vi "SetMeasurement.vi"(1 "int32DeviceNumber":i32, 2 "MeassurementSettings":T3, 3 "FilterSettings":T2, 4 "TriggerSettings":T1) -> (0 "success":i32)   [LabVIEW 2009]
panel:
  in  "measurementFlag":u32
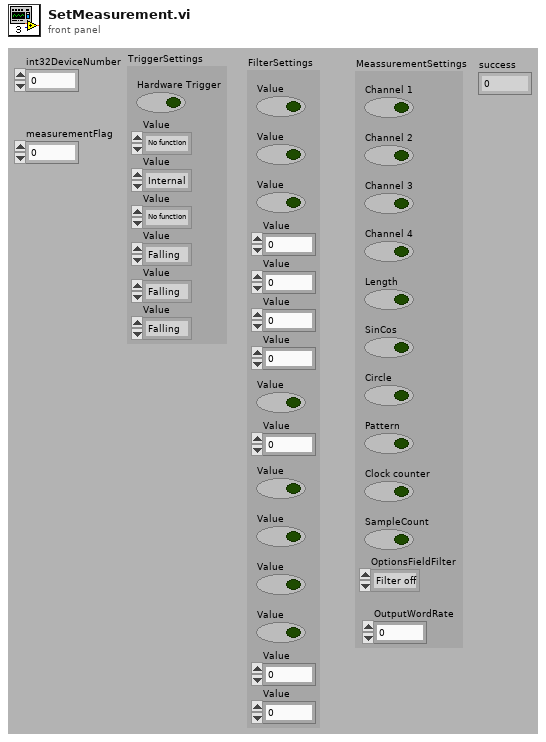
[diagram p1: front panel]
types:
  T1 = cluster{"Hardware Trigger":bool, "Value":enum32{"No function", "Start trigger", "Start/Stop trigger", "Start/Stop processed"}, "Value":enum32{"Internal", "External"}, "Value":enum32{"No function", "Single value"}, "Value":enum32{"Falling", "Rising"}, "Value":enum32{"Falling", "Rising"}, "Value":enum32{"Falling", "Rising"}}
  T2 = cluster{"Value":bool, "Value":bool, "Value":bool, "Value":dbl, "Value":dbl, "Value":dbl, "Value":dbl, "Value":bool, "Value":dbl, "Value":bool, "Value":bool, "Value":bool, "Value":bool, "Value":u8, "Value":u8}
  T3 = cluster{"Channel 1":bool, "Channel 2":bool, "Channel 3":bool, "Channel 4":bool, "Length":bool, "SinCos":bool, "Circle":bool, "Pattern":bool, "Clock counter":bool, "SampleCount":bool, "OptionsFieldFilter":enum32{"Filter off", "Filter default", "Filter user specified"}, "OutputWordRate":dbl}
  T4 = enum32{"Filter off", "Filter default", "Filter user specified"}
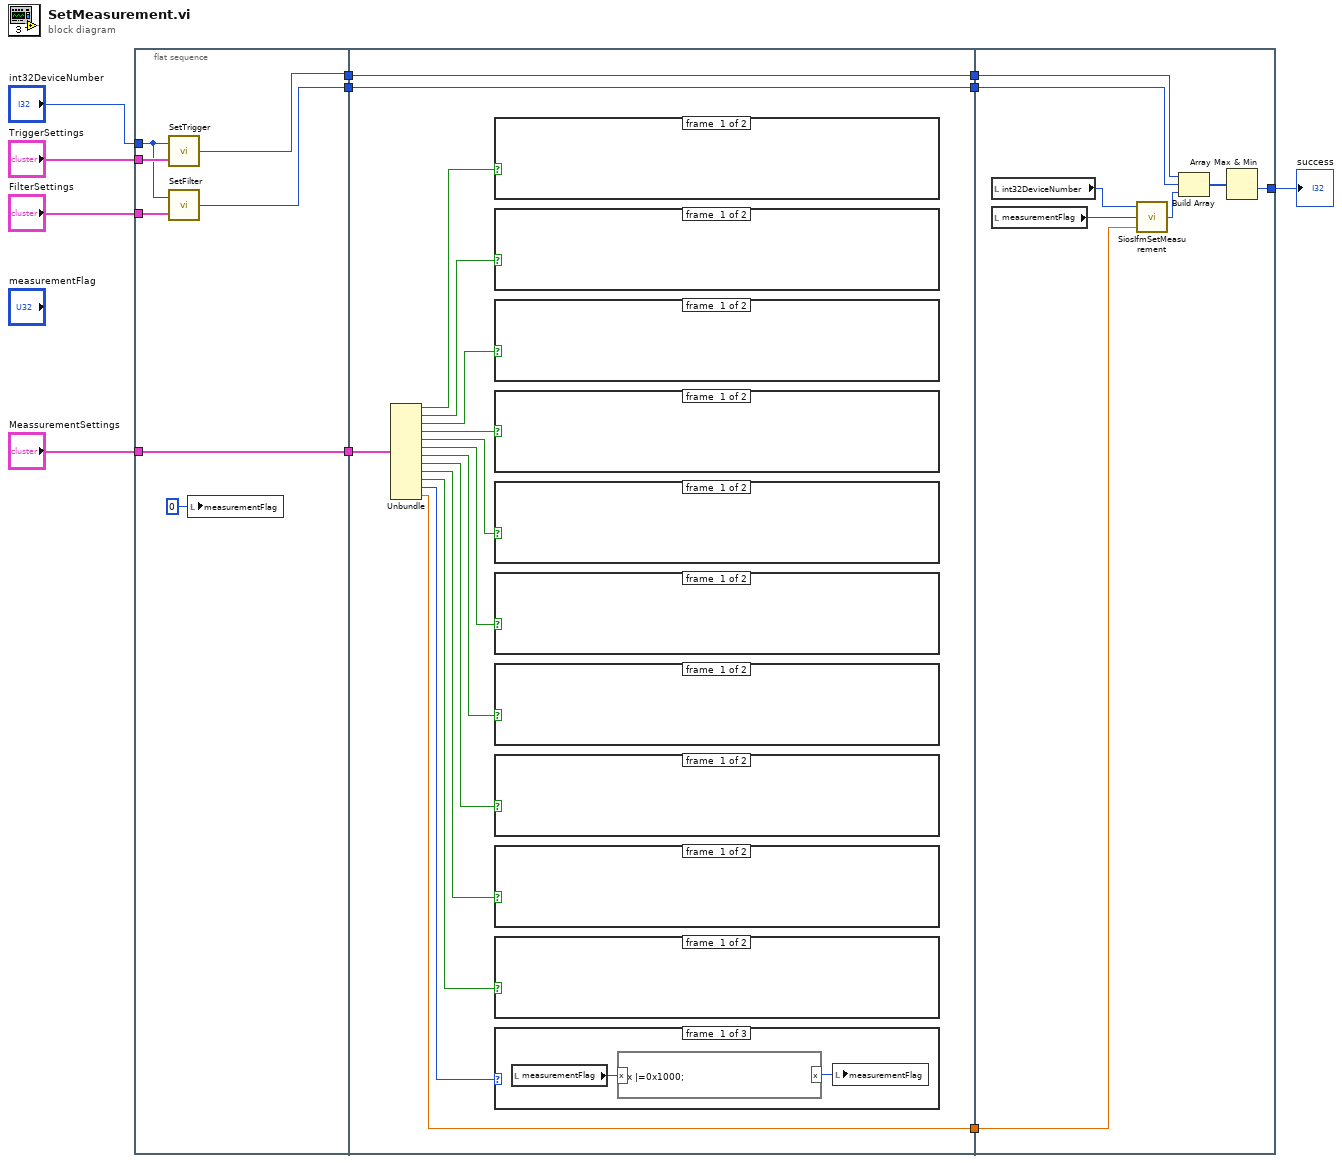
[diagram p0: block diagram]
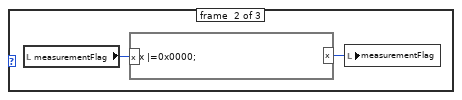
[diagram p2: hidden frame]
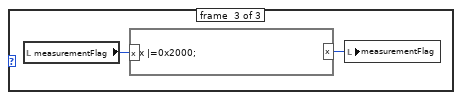
[diagram p3: hidden frame]
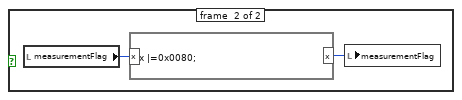
[diagram p4: hidden frame]
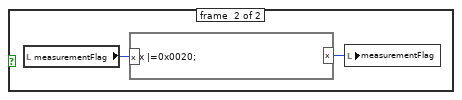
[diagram p5: hidden frame]
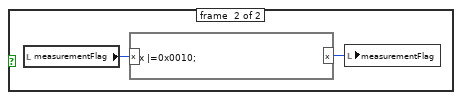
[diagram p6: hidden frame]
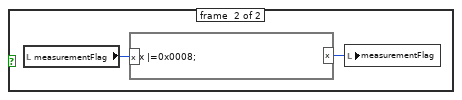
[diagram p7: hidden frame]
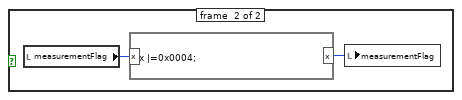
[diagram p8: hidden frame]
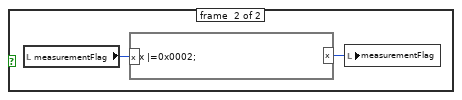
[diagram p9: hidden frame]
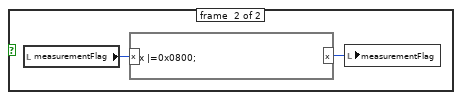
[diagram p10: hidden frame]
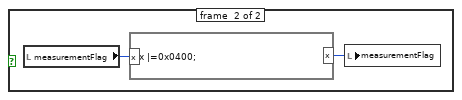
[diagram p11: hidden frame]
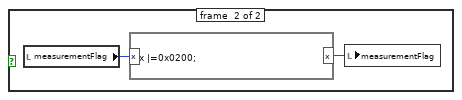
[diagram p12: hidden frame]
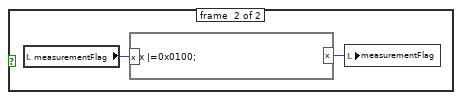
[diagram p13: hidden frame]
diagram:
  n1 = flat-sequence {
    tunnel: "TriggerSettings" -> [w18]
    tunnel: "FilterSettings" -> [w17]
    tunnel: "int32DeviceNumber" -> [w16]
    tunnel: [w15] -> w11
    tunnel: "MeassurementSettings" -> [w15]
    tunnel: [w13] -> w4
    tunnel: [w12] -> w2
    tunnel: w11 -> [w33]
    tunnel: [w21] -> w5
    tunnel: w4 -> [w20]
    tunnel: [w20] -> w3
    tunnel: w2 -> [w19]
    tunnel: [w19] -> w1
    tunnel: [w62] -> w6
    tunnel: w5 -> [w65]
    tunnel: w3 -> [w61]
    tunnel: w1 -> [w60]
    frame #0 {
      n2 = call "SetTrigger.vi"("TriggerSettings"=w18, "deviceNumber"=w16) -> ("success"=w12:i32)
      n3 = call "SetFilter.vi"("FilterSettings"=w17, "DeviceNumber"=w16) -> ("success"=w13:i32)
      n4 = local write "measurementFlag"(u32 0 ("measurementFlag")) -> ()
    }
    frame #1 {
      n5 = Unbundle(w33) -> ("Channel 1"=w32:bool, "Channel 2"=w31:bool, "Channel 3"=w30:bool, "Channel 4"=w29:bool, "Length"=w28:bool, "SinCos"=w27:bool, "Circle"=w26:bool, "Pattern"=w25:bool, "Clock counter"=w24:bool, "SampleCount"=w23:bool, "OptionsFieldFilter"=w22:T4, "OutputWordRate"=w21:dbl)
      n6 = case shown="True" w32 {
        frame #0 {
        }
        frame #1 {
          n7 = local read "measurementFlag"() -> (w58:u32)
          n8 = formula code="x |=0x0100;"("x"=w58) -> ("x"=w59:u32)
          n9 = local write "measurementFlag"(w59) -> ()
        }
      }
      n10 = case shown="True" w31 {
        frame #0 {
        }
        frame #1 {
          n11 = local read "measurementFlag"() -> (w56:u32)
          n12 = formula code="x |=0x0200;"("x"=w56) -> ("x"=w57:u32)
          n13 = local write "measurementFlag"(w57) -> ()
        }
      }
      n14 = case shown="True" w30 {
        frame #0 {
        }
        frame #1 {
          n15 = local read "measurementFlag"() -> (w54:u32)
          n16 = formula code="x |=0x0400;"("x"=w54) -> ("x"=w55:u32)
          n17 = local write "measurementFlag"(w55) -> ()
        }
      }
      n18 = case shown="True" w29 {
        frame #0 {
        }
        frame #1 {
          n19 = local read "measurementFlag"() -> (w52:u32)
          n20 = formula code="x |=0x0800;"("x"=w52) -> ("x"=w53:u32)
          n21 = local write "measurementFlag"(w53) -> ()
        }
      }
      n22 = case shown="True" w28 {
        frame #0 {
        }
        frame #1 {
          n23 = local read "measurementFlag"() -> (w50:u32)
          n24 = formula code="x |=0x0002;"("x"=w50) -> ("x"=w51:u32)
          n25 = local write "measurementFlag"(w51) -> ()
        }
      }
      n26 = case shown="True" w27 {
        frame #0 {
        }
        frame #1 {
          n27 = local read "measurementFlag"() -> (w48:u32)
          n28 = formula code="x |=0x0004;"("x"=w48) -> ("x"=w49:u32)
          n29 = local write "measurementFlag"(w49) -> ()
        }
      }
      n30 = case shown="True" w26 {
        frame #0 {
        }
        frame #1 {
          n31 = local read "measurementFlag"() -> (w46:u32)
          n32 = formula code="x |=0x0008;"("x"=w46) -> ("x"=w47:u32)
          n33 = local write "measurementFlag"(w47) -> ()
        }
      }
      n34 = case shown="True" w25 {
        frame #0 {
        }
        frame #1 {
          n35 = local read "measurementFlag"() -> (w44:u32)
          n36 = formula code="x |=0x0010;"("x"=w44) -> ("x"=w45:u32)
          n37 = local write "measurementFlag"(w45) -> ()
        }
      }
      n38 = case shown="True" w24 {
        frame #0 {
        }
        frame #1 {
          n39 = local read "measurementFlag"() -> (w42:u32)
          n40 = formula code="x |=0x0020;"("x"=w42) -> ("x"=w43:u32)
          n41 = local write "measurementFlag"(w43) -> ()
        }
      }
      n42 = case shown="True" w23 {
        frame #0 {
        }
        frame #1 {
          n43 = local read "measurementFlag"() -> (w40:u32)
          n44 = formula code="x |=0x0080;"("x"=w40) -> ("x"=w41:u32)
          n45 = local write "measurementFlag"(w41) -> ()
        }
      }
      n46 = case shown="\"Filter off\", Default" w22 {
        frame #0 {
          n47 = local read "measurementFlag"() -> (w34:u32)
          n48 = formula code="x |=0x1000;"("x"=w34) -> ("x"=w35:u32)
          n49 = local write "measurementFlag"(w35) -> ()
        }
        frame #1 {
          n50 = local read "measurementFlag"() -> (w36:u32)
          n51 = formula code="x |=0x0000;"("x"=w36) -> ("x"=w37:u32)
          n52 = local write "measurementFlag"(w37) -> ()
        }
        frame #2 {
          n53 = local read "measurementFlag"() -> (w38:u32)
          n54 = formula code="x |=0x2000;"("x"=w38) -> ("x"=w39:u32)
          n55 = local write "measurementFlag"(w39) -> ()
        }
      }
    }
    frame #2 {
      n56 = local read "int32DeviceNumber"() -> (w67:i32)
      n57 = local read "measurementFlag"() -> (w66:u32)
      n58 = call "SiosIfmSetMeasurement.vi"("OutputWordRate"=w65, "measurementFlag"=w66, "int32DeviceNumber"=w67) -> ("success"=w64:i32)
      n59 = Build Array(w60, w61, w64) -> (w63:i32[])
      n60 = Array Max & Min(array=w63) -> (min value=w62:i32)  [unwired: 3 out]
    }
  }
  "success" <- w6
